vi "niFPGA U32xU16 - MSB.vi"(2 "A":u32, 3 "B":u16) -> (7 "A*B [Hi I32]":u32=2838 format="%08x")   [LabVIEW 2017]
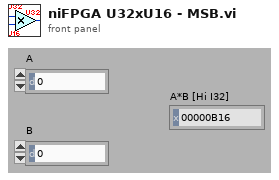
[diagram p1: front panel]
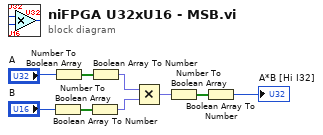
[diagram p0: block diagram]
diagram:
  n1 = Number To Boolean Array(number="B") -> (Boolean array=w5:bool[])
  n2 = Number To Boolean Array(number="A") -> (Boolean array=w4:bool[])
  n3 = Boolean Array To Number(Boolean array=w5) -> (number=w6:fxp<+,16,0>)
  n4 = Boolean Array To Number(Boolean array=w4) -> (number=w7:fxp<+,32,0>)
  n5 = Multiply(x=w7, y=w6) -> (x*y=w9:fxp<+,32,0>)
  n6 = Number To Boolean Array(number=w9) -> (Boolean array=w8:bool[])
  n7 = Boolean Array To Number(Boolean array=w8) -> (number=→"A*B [Hi I32]":u32)
